vi "TTM Get Message.vi"() -> (0 "Text":string, 1 "TTM Message Type":T1(ring))   [LabVIEW 2010]
panel:
  in  "Timeout":i32=-1
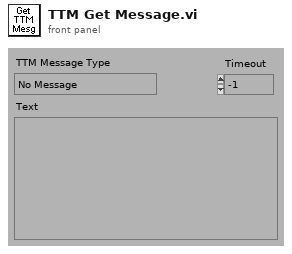
[diagram p1: front panel]
types:
  T1 = enum16{"No Message", "Bad Message", "He3Range=", "He4Range=", "GenEvent=", "Ping=", "Stop"}
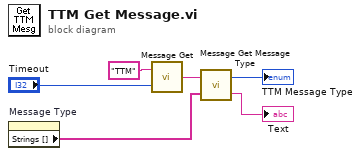
[diagram p0: block diagram]
diagram:
  n1 = property on="Message Type" class="Enum (strict)"() -> ("Strings []"=w3:string[])  [unwired: 2 in, 2 out]
  n2 = call "Message Get.vi"("Timeout ms (-1)"="Timeout", "Module"="TTM") -> ("data out"=w5:string)
  n3 = call "Message Get Message Type.vi"("Message Types"=w3, "Message"=w5) -> ("Trailing text"=→"Text":string, "Message Type"=→"TTM Message Type":i32)
